vi "Check if Valid and Generate Error.vi"(5 "generate error if invalid (F)":bool, 7 "chain levels to remove (2)":i32=2, 8 "error in (no error)":errorcluster, 11 "sentence":string) -> (0 "error out":errorcluster, 3 "valid sentence":bool)   [LabVIEW 2024]
panel:
  in  "<append> (\"\")":string
  in  "<err> (\"\")":string
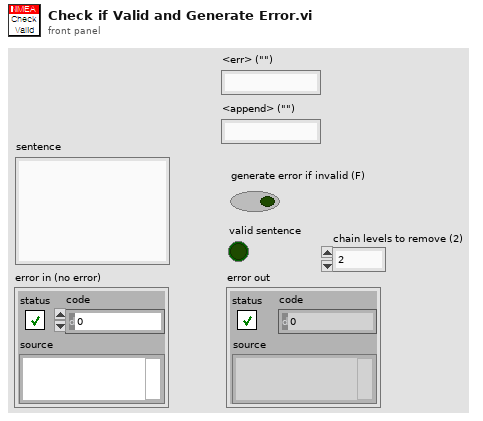
[diagram p1: front panel]
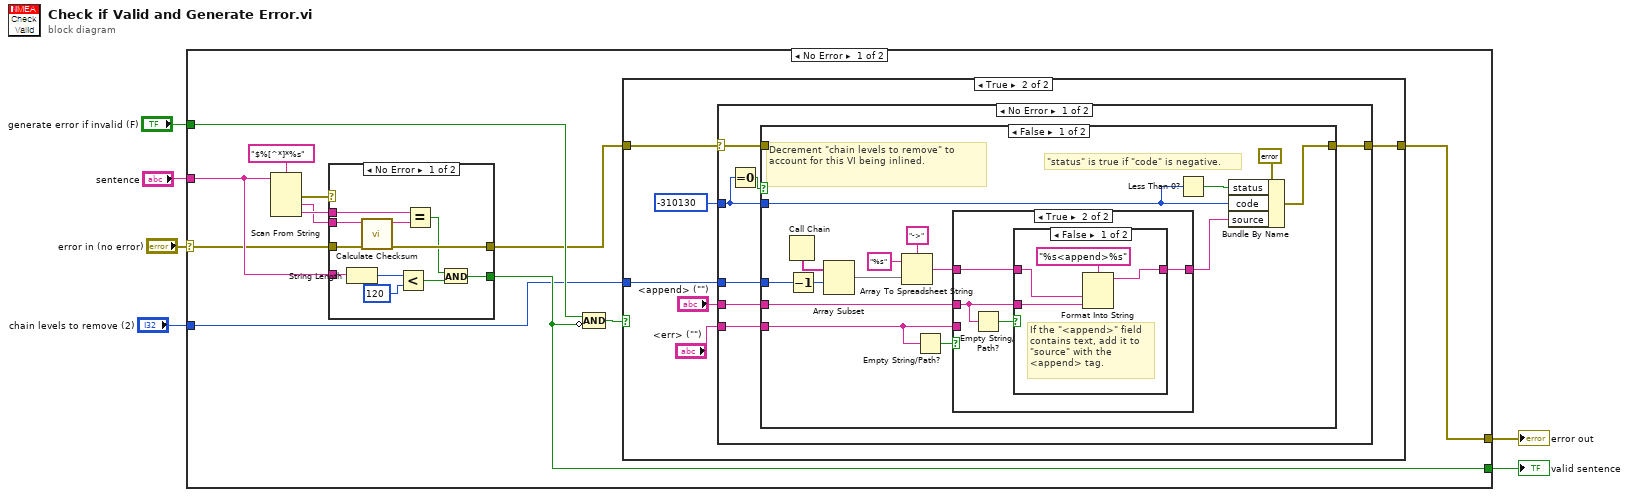
[diagram p0: block diagram]
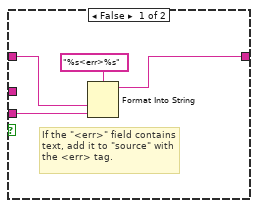
[diagram p3: hidden frame]
diagram:
  n1 = case shown="No Error" "error in (no error)" {
    selector: "error in (no error)" -> [w13 w75]
    tunnel: "sentence" -> [w16 _]
    tunnel: [w7 w75] -> w3
    tunnel: [w11 _] -> w4
    tunnel: "generate error if invalid (F)" -> [w12 _]
    tunnel: "chain levels to remove (2)" -> [w8 _]
    frame No Error {
      n2 = Scan From String(format string="$%[^*]*%s", input string=w16) -> (error out=w14:errorcluster, output 1=w15:string, output 2=w17:string)  [unwired: 2 in, 4 out]
      n3 = case shown="No Error" w14 {
        tunnel: w17 -> [w73 _]
        tunnel: w16 -> [w72 _]
        tunnel: [w64 _] -> w11
        tunnel: w15 -> [w63 _]
        tunnel: [w68 w74] -> w9
        tunnel: w13 -> [w67 w74]
        frame No Error {
          n4 = String Length(string=w72) -> (length=w71:i32)
          n5 = call "Calculate Checksum.vi"("error in (no error)"=w67, "string"=w63) -> ("error out"=w68:errorcluster, "checksum"=w69:string)  [unwired: 8 in]
          n6 = Less?(x=w71, y=120) -> (x < y?=w66:bool)
          n7 = Equal?(x=w73, y=w69) -> (x = y?=w65:bool)
          n8 = And(x=w65, y=w66) -> (x .and. y?=w64:bool)
        }
        frame Error {
        }
      }
      n9 = Compound Arithmetic op=AND(w12, invert w11) -> (w10:bool)
      n10 = case shown="True" w10 {
        tunnel: w9 -> [w19 w23]
        tunnel: w8 -> [_ w21]
        tunnel: [w19 w20] -> w7
        frame False {
        }
        frame True {
          n11 = case shown="No Error" w23 {
            selector: w23 -> [w30 w62]
            tunnel: [w31 w62] -> w20
            tunnel: -310130 ("code") -> [w29 _]
            tunnel: w21 -> [w32 _]
            tunnel: "<err> (\"\")" -> [w28 _]
            tunnel: "<append> (\"\")" -> [w27 _]
            frame No Error {
              n12 = Equal To 0?(x=w29) -> (x = 0?=w26:bool)
              n13 = case shown="False" w26 {
                tunnel: w30 -> [_ w61]
                tunnel: w32 -> [w46 _]
                tunnel: [w44 w61] -> w31
                tunnel: w29 -> [w40 _]
                tunnel: w28 -> [w37 _]
                tunnel: w27 -> [w36 _]
                frame False {
                  # "Decrement \"chain levels to remove\" to account for this VI being inlined."
                  # "\"status\" is true if \"code\" is negative."
                  n14 = Call Chain() -> (call chain=w47:string[])
                  n15 = Decrement(x=w46) -> (x-1=w33:i32)
                  n16 = Array Subset(array=w47, index=w33) -> (w43:string[])  [unwired: 1 in]
                  n17 = Array To Spreadsheet String(delimiter (Tab)="->", array=w43, 3:"%s" ("format string")) -> (spreadsheet string=w39:string)
                  n18 = Empty String/Path?(string/path=w37) -> (empty?=w38:bool)
                  n19 = case shown="True" w38 {
                    tunnel: w39 -> [w48 w53]
                    tunnel: w37 -> [w49 _]
                    tunnel: w36 -> [_ w54]
                    tunnel: [w50 w52] -> w35
                    frame False {
                      # "If the \"<err>\" field contains text, add it to \"source\" with the <err> tag."
                      n20 = Format Into String(format string="%s<err>%s", w48, w49) -> (resulting string=w50:string)  [unwired: 2 in, 1 out]
                    }
                    frame True {
                      n21 = Empty String/Path?(string/path=w54) -> (empty?=w55:bool)
                      n22 = case shown="False" w55 {
                        tunnel: w54 -> [w58 _]
                        tunnel: w53 -> [w59 w60]
                        tunnel: [w56 w60] -> w52
                        frame False {
                          # "If the \"<append>\" field contains text, add it to \"source\" with the <append> tag."
                          n23 = Format Into String(format string="%s<append>%s", w59, w58) -> (resulting string=w56:string)  [unwired: 2 in, 1 out]
                        }
                        frame True {
                        }
                      }
                    }
                  }
                  n24 = Less Than 0?(x=w40) -> (x < 0?=w45:bool)
                  n25 = Bundle By Name(cluster=errorcluster {"status"=FALSE, "code"=0, "source"=""} ("error IO"), "status"=w45, "code"=w40, "source"=w35) -> (w44:errorcluster)
                }
                frame True {
                  # "Do nothing if the new code is zero."
                }
              }
            }
            frame Error {
              # "Do nothing if there is already an error on the wire."
            }
          }
        }
      }
    }
    frame Error {
    }
  }
  "valid sentence" <- w4
  "error out" <- w3
